vi "Start Measurements.vi"(6 "Reply to":refnum<class "Result Reply Msg.lvclass">, 7 "Objects enqueuers":refnum<class "Message Enqueuer.lvclass">[](array[class]), 8 "error in (no error)":errorcluster, 10 "Objects":string[](array[string]), 11 "Pulse Controller in":refnum<class "Pulse Controller.lvclass">) -> (0 "error out":errorcluster, 3 "Pulse Controller out":refnum<class "Pulse Controller.lvclass">)   [LabVIEW 2015, in "Pulse Controller.lvclass"]
uses:
  Pulse Controller.lvclass
  Measure Object Messages/Result Reply Msg/Result Reply Msg.lvclass
  <vilib>/ActorFramework/Message Enqueuer/Message Enqueuer.lvclass
  Pulse Controller.lvclass/Pulse Controller.ctl
  Measure Controller/Measure Controller.lvclass
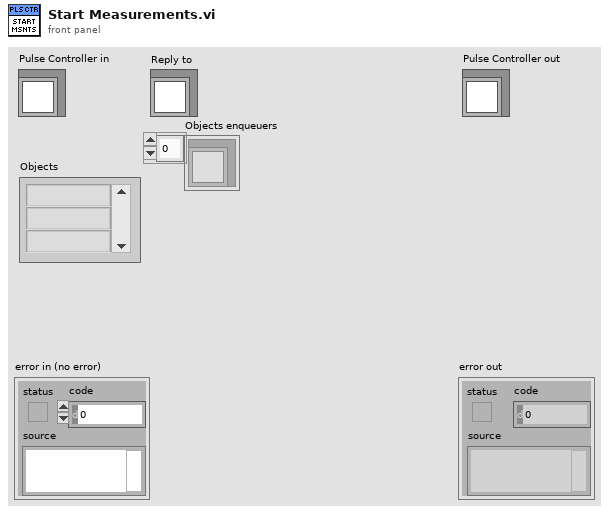
[diagram p1: front panel]
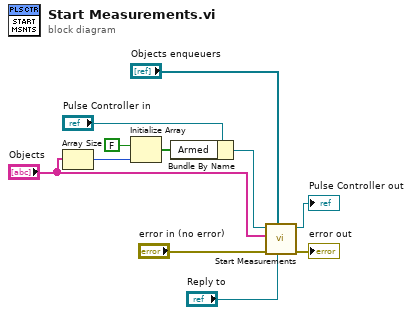
[diagram p0: block diagram]
diagram:
  n1 = Array Size(array="Objects") -> (size(s)=w2:i32)
  n2 = Initialize Array(FALSE, w2) -> (w1:bool[])
  n3 = Bundle By Name(cluster="Pulse Controller in", "Armed"=w1) -> (w5:refnum<class "Pulse Controller.lvclass">)
  n4 = call-parent "Start Measurements.vi"("Reply to"="Reply to", "Objects enqueuers"="Objects enqueuers", "error in (no error)"="error in (no error)", "Objects"="Objects", "Measure Controller in"=w5) -> ("error out"=→"error out":errorcluster, "Measure Controller out"=→"Pulse Controller out":refnum<class "Pulse Controller.lvclass">)  [unwired: 5 in]
